vi "Get Acquired Data.vi"(8 "error in (no error)":errorcluster, 11 "CCDCamera in":refnum<class "CCDCamera.lvclass">) -> (0 "error out":errorcluster, 3 "CCDCamera out":refnum<class "CCDCamera.lvclass">)   [LabVIEW 2018, in "CCDCamera.lvclass"]
uses:
  CCDCamera.lvclass
  CCDCamera.lvclass/CCDCamera.ctl
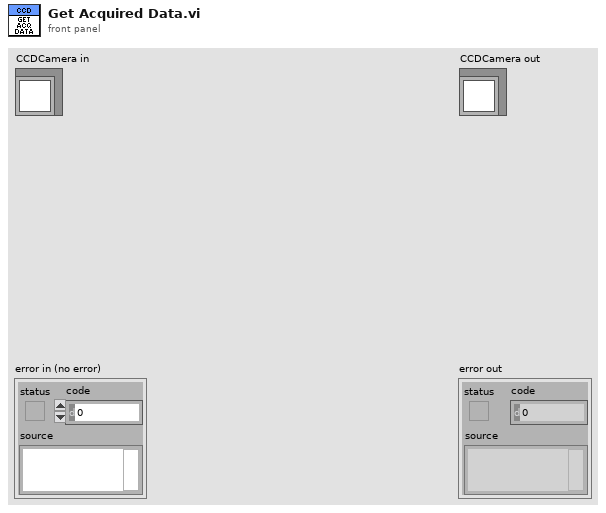
[diagram p1: front panel]
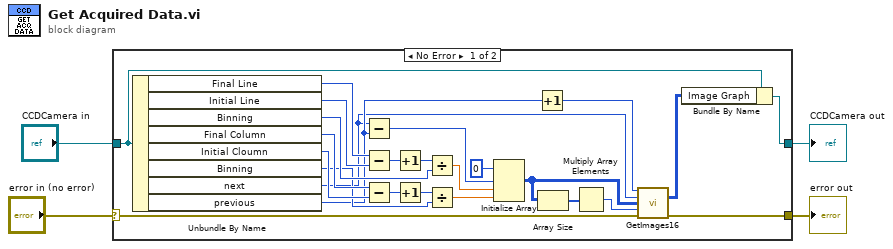
[diagram p0: block diagram]
diagram:
  n1 = case shown="No Error" "error in (no error)" {
    selector: "error in (no error)" -> [w17 w31]
    tunnel: [w16 w31] -> w1
    tunnel: [w29 w30] -> w2
    tunnel: "CCDCamera in" -> [w7 w30]
    frame No Error {
      n2 = Unbundle By Name(w7) -> ("Final Line"=w28:u16, "Initial Line"=w27:u16, "Binning"=w21:u16, "Final Column"=w26:u16, "Initial Cloumn"=w25:u16, "Binning"=w19:u16, "next"=w6:u16, "previous"=w8:u16)
      n3 = Subtract(x=w6, y=w8) -> (x-y=w10:u16)
      n4 = Subtract(x=w28, y=w27) -> (x-y=w24:u16)
      n5 = Subtract(x=w26, y=w25) -> (x-y=w23:u16)
      n6 = Increment(x=w24) -> (x+1=w22:u16)
      n7 = Increment(x=w23) -> (x+1=w20:u16)
      n8 = Divide(x=w22, y=w21) -> (x/y=w15:dbl)
      n9 = Divide(x=w20, y=w19) -> (x/y=w14:dbl)
      n10 = Initialize Array(u16 0, w10, w15, w14) -> (w13:u16[][][])
      n11 = Increment(x=w8) -> (x+1=w9:u16)
      n12 = Array Size(array=w13) -> (size(s)=w12:i32[])
      n13 = Multiply Array Elements(1:w12) -> (0:w11:i32)
      n14 = call <userlib>:"GetImages16.vi"("first"=w9, "last"=w6, "array"=w13, "size"=w11, "error in (no error)"=w17) -> ("array"=w5:u16[][][], "error out"=w16:errorcluster)  [unwired: 6 in, 3 out]
      n15 = Bundle By Name(cluster=w7, "Image Graph"=w5) -> (w29:refnum<class "CCDCamera.lvclass">)
    }
    frame Error {
    }
  }
  "error out" <- w1
  "CCDCamera out" <- w2
